vi "GetCoeffsAndComp.vi"(10 "mutedData":dbl[](array[numeric])) -> (2 "boostedData":dbl[](array[numeric]))   [LabVIEW 2011]
uses:
  Globals/Meas_global.vi
  Globals/Constants_global.vi
panel:
  out "TubingCorrectionFile (pre-set!)":path
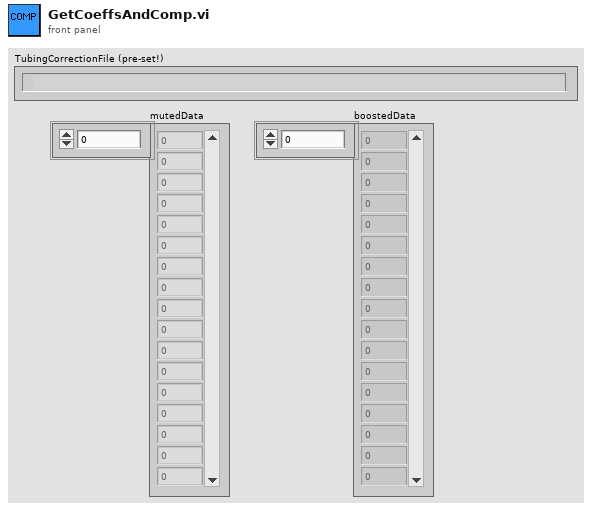
[diagram p1: front panel]
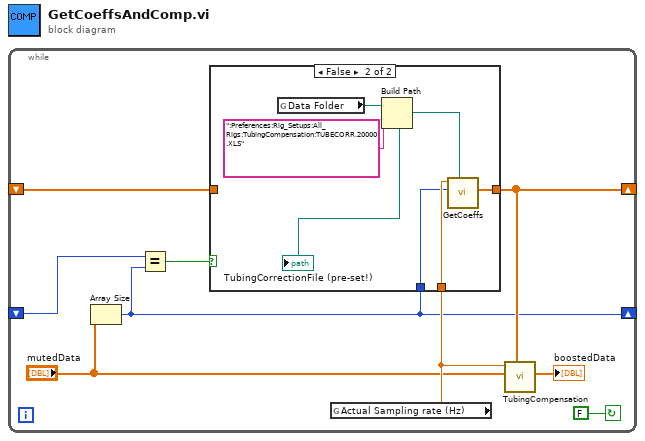
[diagram p0: block diagram]
diagram:
  n1 = while {
    shift-right: [w8] -> _
    shift-left: _ -> [w9]
    shift-right: [w2] -> _
    shift-left: _ -> [w1]
    stop <- FALSE continue-if-true
    n2 = Array Size(array="mutedData") -> (size(s)=w2:i32)
    n3 = Equal?(x=w1, y=w2) -> (x = y?=w4:bool)
    n4 = global read "Meas_global.vi" "Actual Sampling rate (Hz)"() -> (w5:dbl)
    n5 = case shown="False" w4 {
      tunnel: [w10 w16] -> w8
      tunnel: w9 -> [w10 _]
      tunnel: w5 -> [_ w15]
      tunnel: w2 -> [_ w11]
      frame True {
      }
      frame False {
        n6 = global read "Constants_global.vi" "Data Folder"() -> (w14:path)
        n7 = Build Path(base path=w14, name or relative path=":Preferences:Rig_Setups:All_Rigs:TubingCompensation:TUBECORR.20000.XLS") -> (appended path=w13:path)
        "TubingCorrectionFile (pre-set!)" <- w13
        n8 = call "GetCoeffs.vi"("PathToFile"=w13, "SignalLength"=w11, "fs (Hz)"=w15) -> ("NyquistLimitedCoefficients"=w16:dbl[])  [unwired: 8 in]
      }
    }
    n9 = call "TubingCompensation.vi"("NyquistLimitedCoefficients"=w8, "mutedData"="mutedData", "SamplingFreq"=w5) -> ("boostedData"=→"boostedData":dbl[])  [unwired: 8 in]
  }
